vi "ExampleStateMachine-CalculatorEvents.vi"() -> ()   [LabVIEW 2017]
panel:
  in  "ADD":bool
  in  "SUB":bool
  in  "MULT":bool
  in  "DIV":bool
  in  "CLR":bool
  in  "Number 2":dbl=2.0
  in  "Number 1":dbl=4.0
  out "Result":dbl
  in  "stop":bool
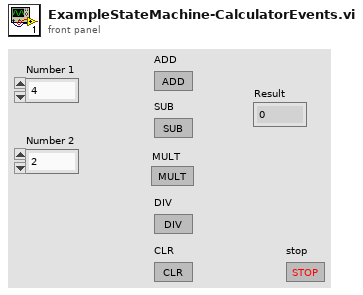
[diagram p1: front panel]
types:
  T1 = enum16{"Initialize", "Wait", "Add", "Subtract", "Multiply", "Divide", "Clear"}
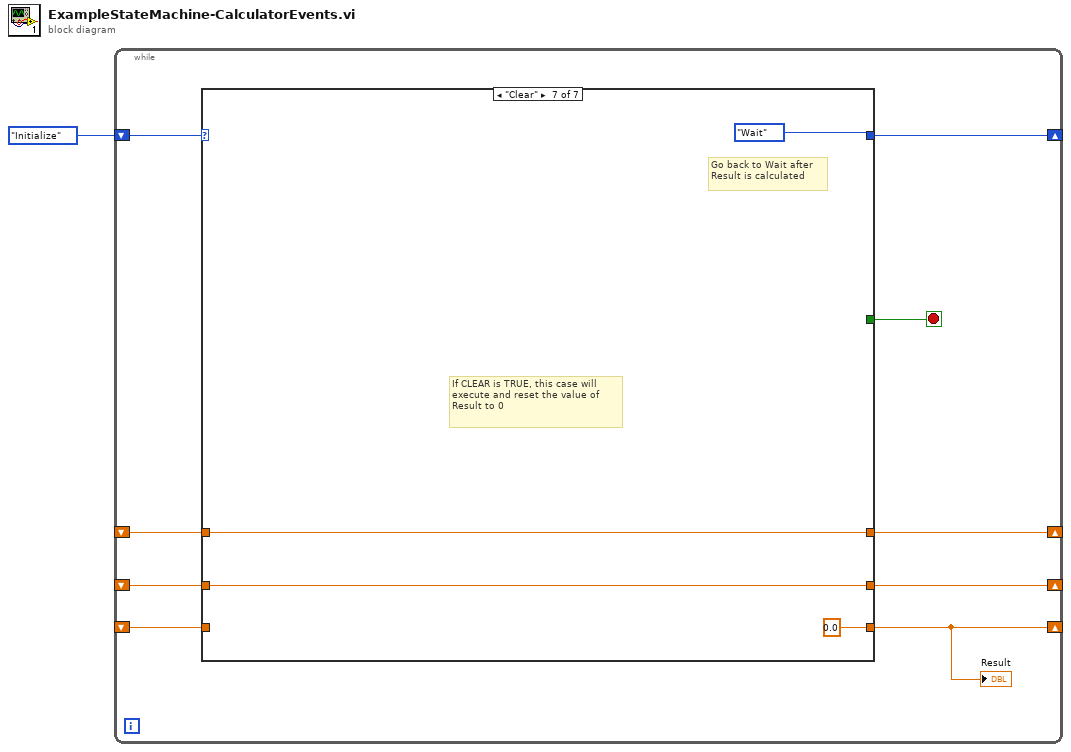
[diagram p0: block diagram]
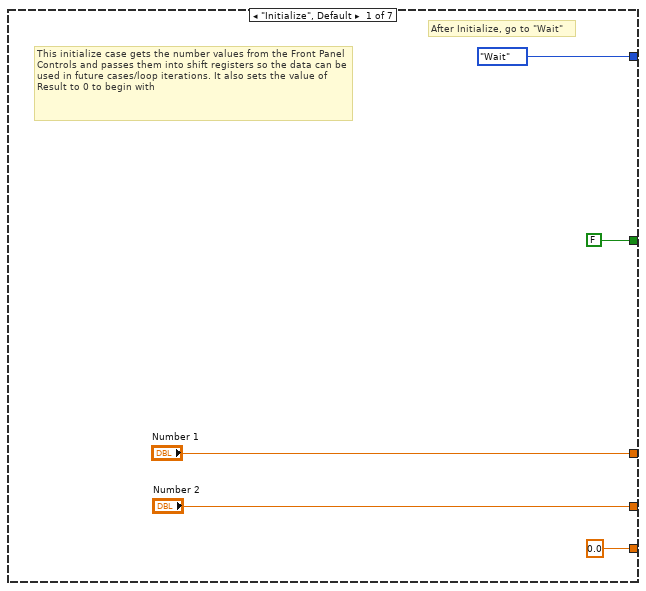
[diagram p2: hidden frame]
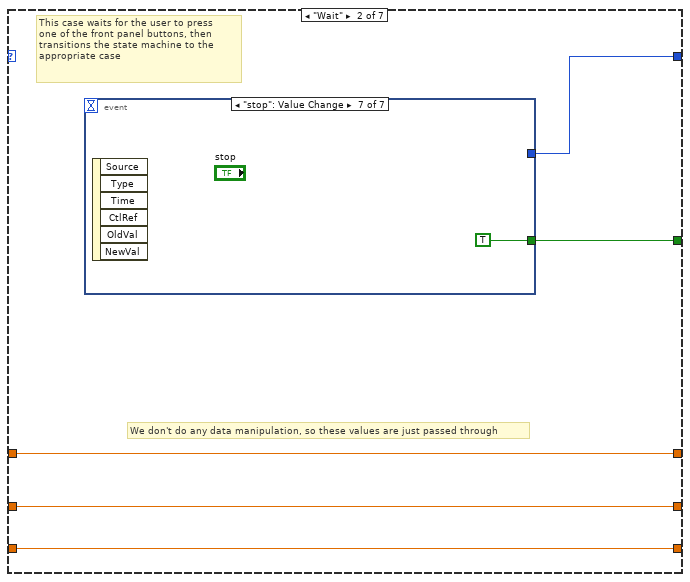
[diagram p3: hidden frame]
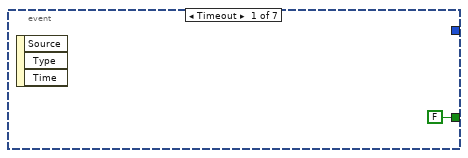
[diagram p4: hidden frame]
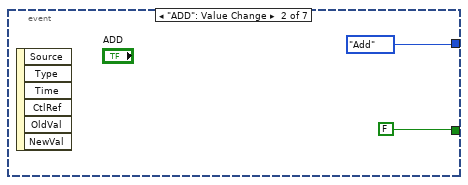
[diagram p5: hidden frame]
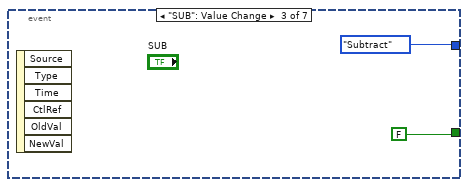
[diagram p6: hidden frame]
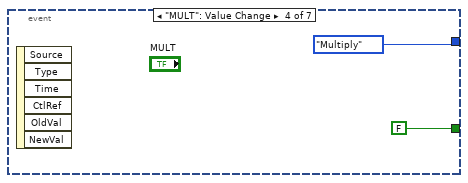
[diagram p7: hidden frame]
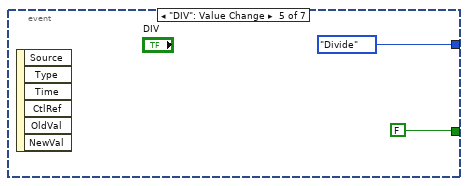
[diagram p8: hidden frame]
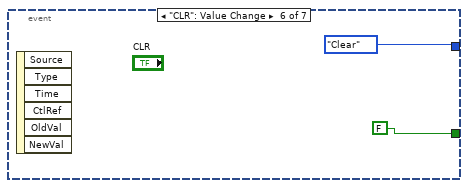
[diagram p9: hidden frame]
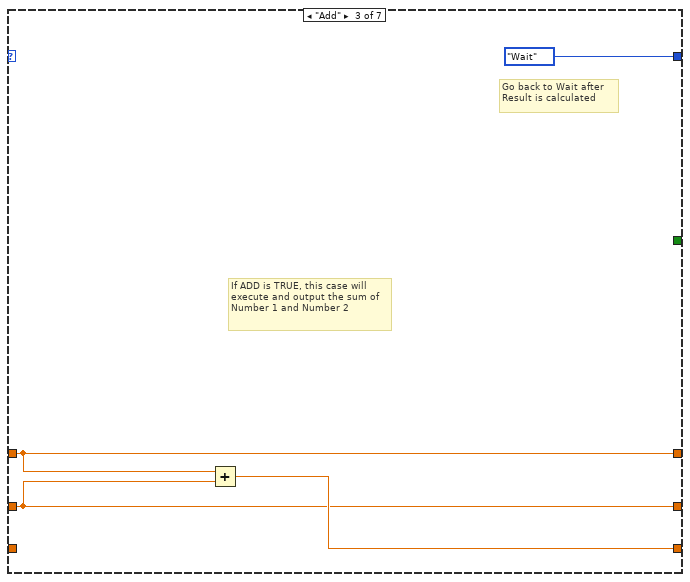
[diagram p10: hidden frame]
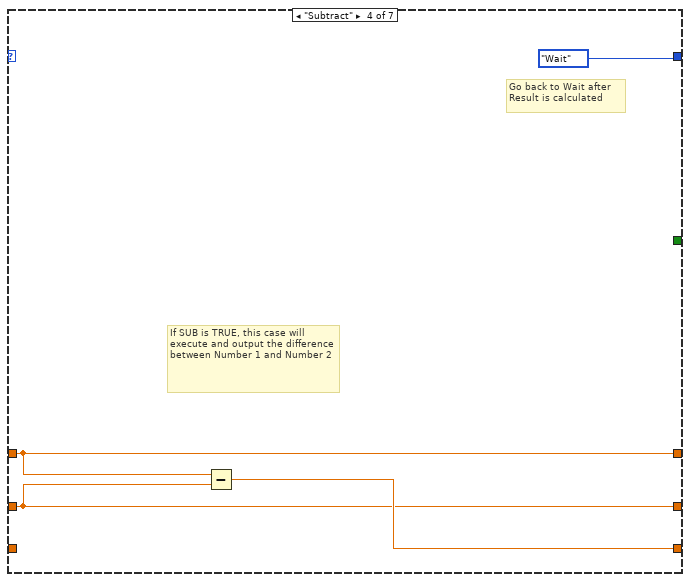
[diagram p11: hidden frame]
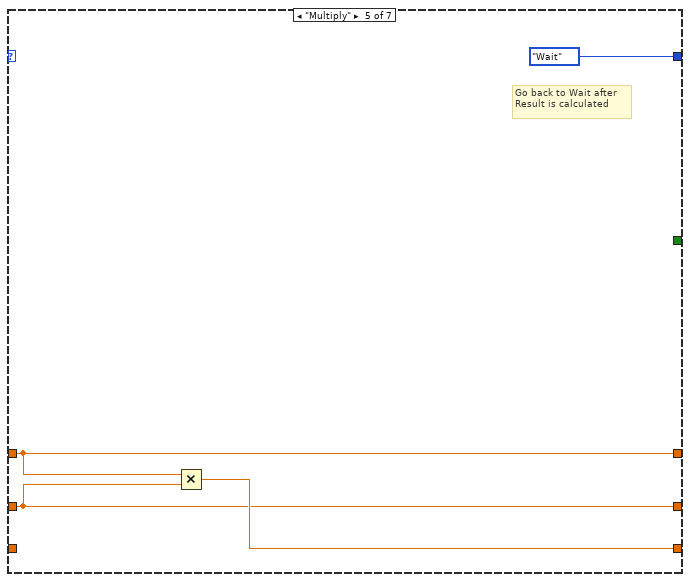
[diagram p12: hidden frame]
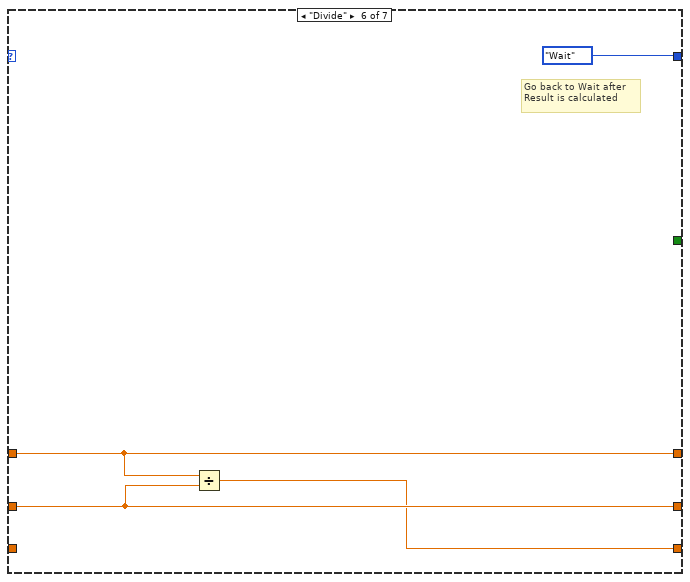
[diagram p13: hidden frame]
diagram:
  n1 = while {
    shift-right: [w9] -> _
    shift-left: _ -> [w6]
    shift-right: [w8] -> _
    shift-left: _ -> [w5]
    shift-right: [w7] -> _
    shift-left: T1."Initialize" -> [w10]
    shift-right: [w4] -> _
    shift-left: _ -> [w3]
    stop <- w2 stop-if-true
    n2 = case shown="\"Clear\"" w10 {
      tunnel: ["Number 1" w20 w34 w39 w43 w48 w51] -> w9
      tunnel: ["Number 2" w19 w33 w38 w42 w47 w50] -> w8
      tunnel: [T1."Wait" w17 T1."Wait" T1."Wait" T1."Wait" T1."Wait" T1."Wait"] -> w7
      tunnel: w6 -> [_ w20 w34 w39 w43 w48 w51]
      tunnel: w5 -> [_ w19 w33 w38 w42 w47 w50]
      tunnel: [0.0 w18 w35 w40 w44 w46 0.0] -> w4
      tunnel: w3 -> [_ w18 _ _ _ _ _]
      tunnel: [FALSE w16 _ _ _ _ _] -> w2
      frame "Initialize", Default {
        # "After Initialize, go to \"Wait\""
        # "This initialize case gets the number values from the Front Panel Controls and passes them into shift registers so the data can be used in future cases/loop iterations. It also sets the value of Result to 0 to begin with"
      }
      frame "Wait" {
        # "We don't do any data manipulation, so these values are just passed through"
        # "This case waits for the user to press\none of the front panel buttons, then\ntransitions the state machine to the \nappropriate case"
        n3 = event shown="[6] \"stop\": Value Change" {
          selector: _ -> [_ _ _ _ _ _ _]
          dyn-events: _ -> [_ _ _ _ _ _ _]
          timeout: _ -> [_ _ _ _ _ _ _]
          tunnel: [_ T1."Add" T1."Subtract" T1."Multiply" T1."Divide" T1."Clear" _] -> w17
          tunnel: [FALSE FALSE FALSE FALSE FALSE FALSE TRUE] -> w16
          event Timeout {
            n4 = event-data() -> ()  [unwired: 1 in, 3 out]
          }
          event "ADD": Value Change {
            n5 = event-data() -> ()  [unwired: 1 in, 6 out]
          }
          event "SUB": Value Change {
            n6 = event-data() -> ()  [unwired: 1 in, 6 out]
          }
          event "MULT": Value Change {
            n7 = event-data() -> ()  [unwired: 1 in, 6 out]
          }
          event "DIV": Value Change {
            n8 = event-data() -> ()  [unwired: 1 in, 6 out]
          }
          event "CLR": Value Change {
            n9 = event-data() -> ()  [unwired: 1 in, 6 out]
          }
          event "stop": Value Change {
            n10 = event-data() -> ()  [unwired: 1 in, 6 out]
          }
        }
      }
      frame "Add" {
        # "Go back to Wait after Result is calculated"
        # "If ADD is TRUE, this case will execute and output the sum of Number 1 and Number 2"
        n11 = Add(x=w34, y=w33) -> (x+y=w35:dbl)
      }
      frame "Subtract" {
        # "Go back to Wait after Result is calculated"
        # "If SUB is TRUE, this case will execute and output the difference between Number 1 and Number 2"
        n12 = Subtract(x=w39, y=w38) -> (x-y=w40:dbl)
      }
      frame "Multiply" {
        # "Go back to Wait after Result is calculated"
        n13 = Multiply(x=w43, y=w42) -> (x*y=w44:dbl)
      }
      frame "Divide" {
        # "Go back to Wait after Result is calculated"
        n14 = Divide(x=w48, y=w47) -> (x/y=w46:dbl)
      }
      frame "Clear" {
        # "Go back to Wait after Result is calculated"
        # "If CLEAR is TRUE, this case will execute and reset the value of Result to 0"
      }
    }
    "Result" <- w4
  }
